vi "Channel VState.vi"(8 "error in (no error)":errorcluster, 11 "VISA resource name":refnum<visa-resource-name>="DSOS404") -> (0 "error out":errorcluster, 2 "Channel Index":cluster{bool, bool, bool, bool}, 3 "VISA resource name 2":refnum<visa-resource-name>)   [LabVIEW 2018]
panel:
  # "CH1"
  # "CH2"
  # "CH3"
  # "CH4"
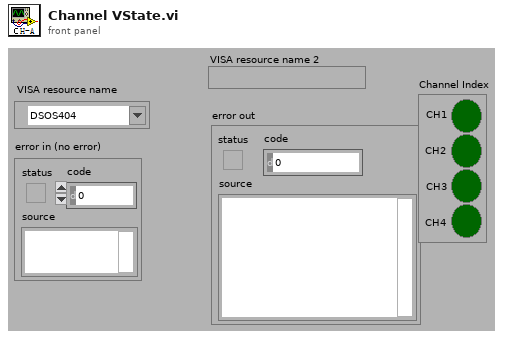
[diagram p1: front panel]
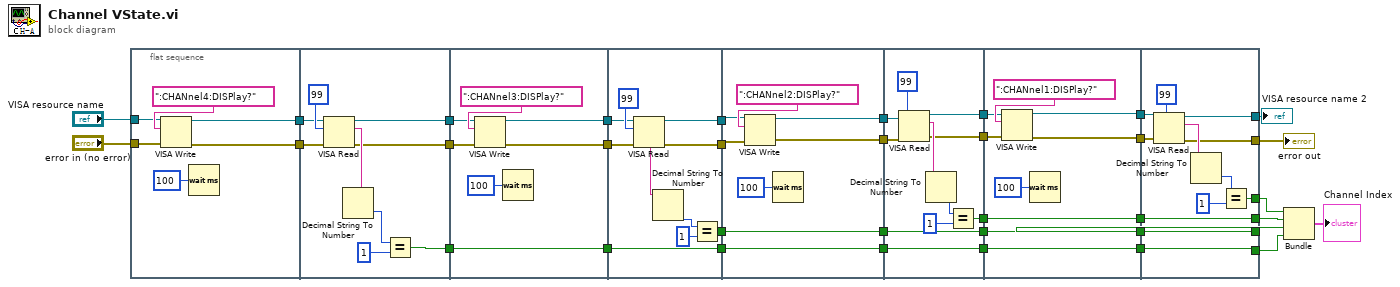
[diagram p0: block diagram]
diagram:
  n1 = flat-sequence {
    tunnel: "VISA resource name" -> [w39]
    tunnel: "error in (no error)" -> [w38]
    tunnel: [w37] -> w33
    tunnel: [w36] -> w32
    tunnel: w33 -> [w46]
    tunnel: w32 -> [w45]
    tunnel: [w44] -> w31
    tunnel: [w43] -> w30
    tunnel: [w42] -> w29
    tunnel: w31 -> [w55]
    tunnel: w30 -> [w54]
    tunnel: w29 -> [w51]
    tunnel: [w53] -> w28
    tunnel: [w52] -> w27
    tunnel: [w51] -> w8
    tunnel: w28 -> [w63]
    tunnel: w27 -> [w62]
    tunnel: [w61] -> w26
    tunnel: [w60] -> w25
    tunnel: [w59] -> w13
    tunnel: [w58] -> w9
    tunnel: w8 -> [w58]
    tunnel: w26 -> [w73]
    tunnel: w25 -> [w72]
    tunnel: [w71] -> w24
    tunnel: [w70] -> w23
    tunnel: [w69] -> w14
    tunnel: w13 -> [w69]
    tunnel: [w68] -> w10
    tunnel: w9 -> [w68]
    tunnel: w24 -> [w82]
    tunnel: w23 -> [w81]
    tunnel: [w80] -> w22
    tunnel: [w79] -> w21
    tunnel: [w78] -> w17
    tunnel: [w77] -> w15
    tunnel: w14 -> [w77]
    tunnel: [w76] -> w11
    tunnel: w10 -> [w76]
    tunnel: w22 -> [w93]
    tunnel: w21 -> [w92]
    tunnel: [w91] -> w20
    tunnel: [w90] -> w19
    tunnel: [w89] -> w18
    tunnel: w17 -> [w89]
    tunnel: [w88] -> w16
    tunnel: w15 -> [w88]
    tunnel: [w87] -> w12
    tunnel: w11 -> [w87]
    tunnel: w20 -> [w103]
    tunnel: w19 -> [w102]
    tunnel: [w101] -> w2
    tunnel: [w100] -> w5
    tunnel: w18 -> [w100]
    tunnel: [w99] -> w4
    tunnel: w16 -> [w99]
    tunnel: [w98] -> w1
    tunnel: w12 -> [w98]
    tunnel: [w97] -> w6
    tunnel: [w96] -> w7
    frame #0 {
      n2 = VISA Write(VISA resource name=w39, write buffer=":CHANnel4:DISPlay?", error in (no error)=w38) -> (VISA resource name out=w37:refnum<visa-resource-name>, error out=w36:errorcluster)  [unwired: 1 out]
      n3 = Wait (ms)(milliseconds to wait=u32 100) -> ()  [unwired: 1 out]
    }
    frame #1 {
      n4 = VISA Read(VISA resource name=w46, byte count=u32 99, error in (no error)=w45) -> (VISA resource name out=w44:refnum<visa-resource-name>, read buffer=w48:string, error out=w43:errorcluster)  [unwired: 1 out]
      n5 = Decimal String To Number(string=w48) -> (number=w49:i32)  [unwired: 2 in, 1 out]
      n6 = Equal?(x=w49, y=1) -> (x = y?=w42:bool)
    }
    frame #2 {
      n7 = VISA Write(VISA resource name=w55, write buffer=":CHANnel3:DISPlay?", error in (no error)=w54) -> (VISA resource name out=w53:refnum<visa-resource-name>, error out=w52:errorcluster)  [unwired: 1 out]
      n8 = Wait (ms)(milliseconds to wait=u32 100) -> ()  [unwired: 1 out]
    }
    frame #3 {
      n9 = VISA Read(VISA resource name=w63, byte count=u32 99, error in (no error)=w62) -> (VISA resource name out=w61:refnum<visa-resource-name>, read buffer=w67:string, error out=w60:errorcluster)  [unwired: 1 out]
      n10 = Decimal String To Number(string=w67) -> (number=w65:i32)  [unwired: 2 in, 1 out]
      n11 = Equal?(x=w65, y=1) -> (x = y?=w59:bool)
    }
    frame #4 {
      n12 = VISA Write(VISA resource name=w73, write buffer=":CHANnel2:DISPlay?", error in (no error)=w72) -> (VISA resource name out=w71:refnum<visa-resource-name>, error out=w70:errorcluster)  [unwired: 1 out]
      n13 = Wait (ms)(milliseconds to wait=u32 100) -> ()  [unwired: 1 out]
    }
    frame #5 {
      n14 = VISA Read(VISA resource name=w82, byte count=u32 99, error in (no error)=w81) -> (VISA resource name out=w80:refnum<visa-resource-name>, read buffer=w84:string, error out=w79:errorcluster)  [unwired: 1 out]
      n15 = Decimal String To Number(string=w84) -> (number=w86:i32)  [unwired: 2 in, 1 out]
      n16 = Equal?(x=w86, y=1) -> (x = y?=w78:bool)
    }
    frame #6 {
      n17 = VISA Write(VISA resource name=w93, write buffer=":CHANnel1:DISPlay?", error in (no error)=w92) -> (VISA resource name out=w91:refnum<visa-resource-name>, error out=w90:errorcluster)  [unwired: 1 out]
      n18 = Wait (ms)(milliseconds to wait=u32 100) -> ()  [unwired: 1 out]
    }
    frame #7 {
      n19 = VISA Read(VISA resource name=w103, byte count=u32 99, error in (no error)=w102) -> (VISA resource name out=w96:refnum<visa-resource-name>, read buffer=w105:string, error out=w97:errorcluster)  [unwired: 1 out]
      n20 = Decimal String To Number(string=w105) -> (number=w107:i32)  [unwired: 2 in, 1 out]
      n21 = Equal?(x=w107, y=1) -> (x = y?=w101:bool)
    }
  }
  n22 = Bundle(w2, w5, w4, w1) -> (→"Channel Index":cluster{bool, bool, bool, bool})  [unwired: 1 in]
  "VISA resource name 2" <- w7
  "error out" <- w6
